vi "Hw Device list.vi"(8 "error in (no error)":errorcluster) -> (0 "error out":errorcluster, 2 "Device List":T1, 3 "Channel List":T2)   [LabVIEW 2020]
uses:
  <resource>/objmgr/daqmx.rc
  b5ac99f9-5173-4c31-8a28-ef8ad511105c.vi
  fb49c12b-b483-4571-b40d-ecaa8db585a3.vi
  68205be7-741a-4ef4-8ff5-1684b69be710.vi
  1e1b64d9-6d49-45cf-9d80-2436e3cb3542.vi
panel:
  out "DO Cards":tag[](array[tag])
  out "DI Cards":tag[](array[tag])
  out "AO Cards":tag[](array[tag])
  out "AI Cards":tag[](array[tag])
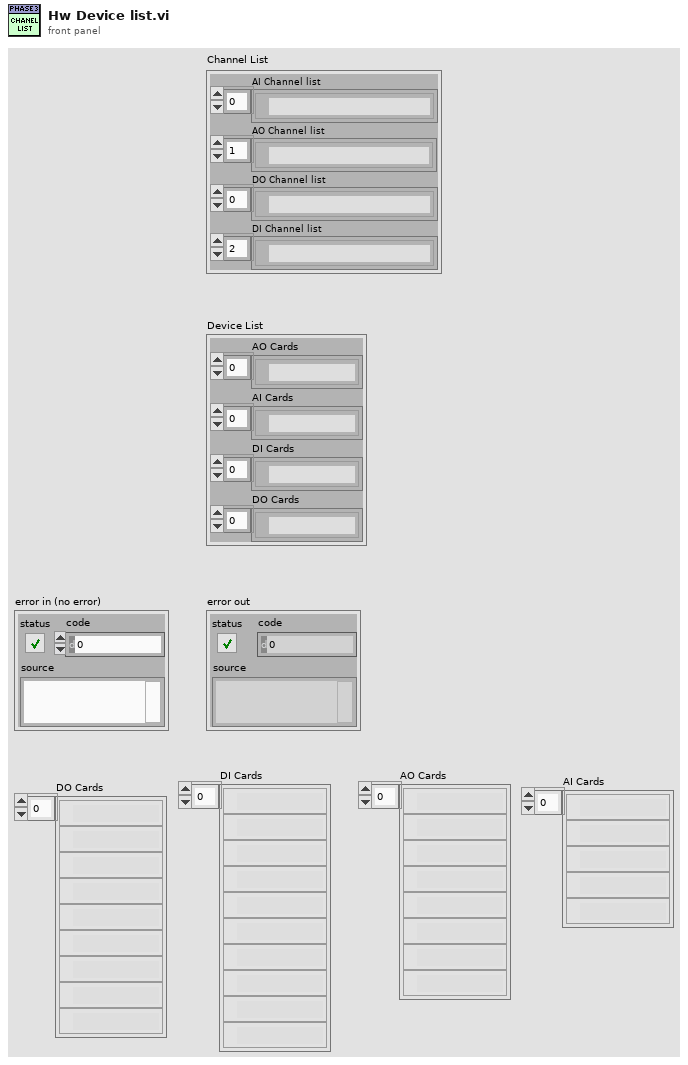
[diagram p1: front panel]
types:
  T1 = cluster{"AO Cards":tag[], "AI Cards":tag[], "DI Cards":tag[], "DO Cards":tag[]}
  T2 = cluster{"AI Channel list":tag[], "AO Channel list":tag[], "DO Channel list ":tag[], "DI Channel list":tag[]}
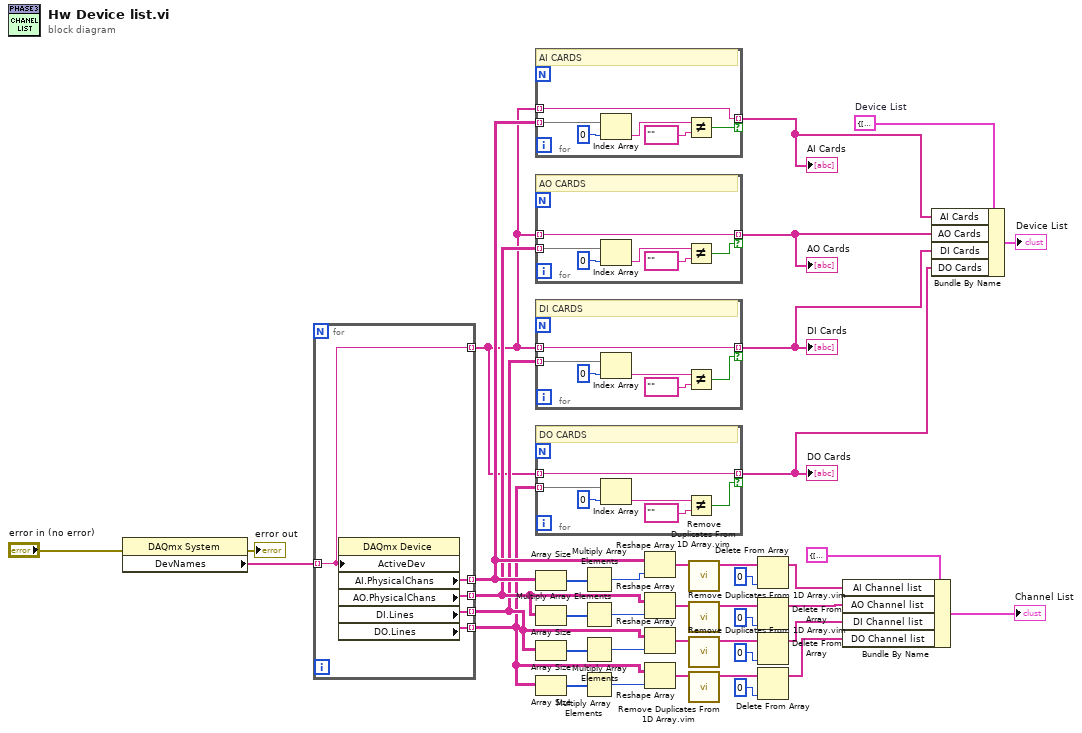
[diagram p0: block diagram]
diagram:
  w7 = T1 {"AO Cards"=[], "AI Cards"=[], "DI Cards"=[], "DO Cards"=[]}  # Device List
  n1 = property class="DAQmx System"(error in="error in (no error)") -> (error out=→"error out":errorcluster, "DevNames"=w40:tag[])  [unwired: 1 in, 1 out]
  n2 = for {
    tunnel: w40 -> [w41] mode=indexing
    tunnel: [w45] -> w11 mode=indexing
    tunnel: [w44] -> w10 mode=indexing
    tunnel: [w43] -> w9 mode=indexing
    tunnel: [w42] -> w8 mode=indexing
    tunnel: [w41] -> w2 mode=indexing
    n3 = property class="DAQmx Device"("ActiveDev"=w41) -> ("AI.PhysicalChans"=w45:tag[], "AO.PhysicalChans"=w44:tag[], "DI.Lines"=w43:tag[], "DO.Lines"=w42:tag[])  [unwired: 2 in, 2 out]
  }
  n4 = for {
    tunnel: w11 -> [w49] mode=indexing
    tunnel: [w51] -> w6 mode=indexing if=w46
    tunnel: w2 -> [w51] mode=indexing
    # "AI CARDS"
    n5 = Index Array(array=w49, index=0) -> (element=w48:tag)
    n6 = Not Equal?(x=w48, y=tag "") -> (x != y?=w46:bool)
  }
  "AI Cards" <- w6
  n7 = for {
    tunnel: w10 -> [w52] mode=indexing
    tunnel: [w57] -> w5 mode=indexing if=w53
    tunnel: w2 -> [w57] mode=indexing
    # "AO CARDS"
    n8 = Index Array(array=w52, index=0) -> (element=w55:tag)
    n9 = Not Equal?(x=w55, y=tag "") -> (x != y?=w53:bool)
  }
  "AO Cards" <- w5
  n10 = for {
    tunnel: w9 -> [w58] mode=indexing
    tunnel: [w63] -> w4 mode=indexing if=w59
    tunnel: w2 -> [w63] mode=indexing
    # "DI CARDS"
    n11 = Index Array(array=w58, index=0) -> (element=w61:tag)
    n12 = Not Equal?(x=w61, y=tag "") -> (x != y?=w59:bool)
  }
  "DI Cards" <- w4
  n13 = for {
    tunnel: w8 -> [w64] mode=indexing
    tunnel: [w69] -> w3 mode=indexing if=w65
    tunnel: w2 -> [w69] mode=indexing
    # "DO CARDS"
    n14 = Index Array(array=w64, index=0) -> (element=w67:tag)
    n15 = Not Equal?(x=w67, y=tag "") -> (x != y?=w65:bool)
  }
  "DO Cards" <- w3
  n16 = Array Size(array=w11) -> (size(s)=w39:i32[])
  n17 = Array Size(array=w10) -> (size(s)=w35:i32[])
  n18 = Array Size(array=w9) -> (size(s)=w31:i32[])
  n19 = Array Size(array=w8) -> (size(s)=w27:i32[])
  n20 = Multiply Array Elements(1:w39) -> (0:w38:i32)
  n21 = Multiply Array Elements(1:w35) -> (0:w34:i32)
  n22 = Multiply Array Elements(1:w31) -> (0:w30:i32)
  n23 = Multiply Array Elements(1:w27) -> (0:w26:i32)
  n24 = Reshape Array(w11, w38) -> (w37:tag[])
  n25 = Reshape Array(w10, w34) -> (w33:tag[])
  n26 = Reshape Array(w9, w30) -> (w29:tag[])
  n27 = Reshape Array(w8, w26) -> (w25:tag[])
  n28 = call "Remove Duplicates From 1D Array.vim"("array"=w37) -> ("array with duplicates removed"=w36:tag[])  [unwired: 10 in]
  n29 = call "Remove Duplicates From 1D Array.vim"("array"=w33) -> ("array with duplicates removed"=w32:tag[])  [unwired: 10 in]
  n30 = call "Remove Duplicates From 1D Array.vim"("array"=w29) -> ("array with duplicates removed"=w28:tag[])  [unwired: 10 in]
  n31 = call "Remove Duplicates From 1D Array.vim"("array"=w25) -> ("array with duplicates removed"=w24:tag[])  [unwired: 10 in]
  n32 = Delete From Array(array=w36, index=0) -> (array with subset deleted=w16:tag[])  [unwired: 1 in, 1 out]
  n33 = Delete From Array(array=w32, index=0) -> (array with subset deleted=w15:tag[])  [unwired: 1 in, 1 out]
  n34 = Delete From Array(array=w28, index=0) -> (array with subset deleted=w14:tag[])  [unwired: 1 in, 1 out]
  n35 = Delete From Array(array=w24, index=0) -> (array with subset deleted=w13:tag[])  [unwired: 1 in, 1 out]
  n36 = Bundle By Name(cluster=T2 {"AI Channel list"=[], "AO Channel list"=[], "DO Channel list "=[], "DI Channel list"=[]} ("Cluster"), "AI Channel list"=w16, "AO Channel list"=w15, "DI Channel list"=w14, "DO Channel list"=w13) -> (→"Channel List":T2)
  n37 = Bundle By Name(cluster=w7, "AI Cards"=w6, "AO Cards"=w5, "DI Cards"=w4, "DO Cards"=w3) -> (→"Device List":T1)
